vi "MPM_Set_Logging_Paremeter_for_STS.vi"(0 ".NET Reference in":refnum<k24>, 1 "startwave":dbl, 2 "stopwave":dbl, 3 "wavestep":dbl, 4 "speed":dbl, 5 "error in (no error)":errorcluster, 7 "mode":i32(ring) items=["ManualRangeConstant", "ManualRangeSweep", "AutoRangeConstant", "AutoRangeSweep", "Freerun"]) -> (14 "Reference out":refnum<k24>, 19 "error out":errorcluster)   [LabVIEW 2017]
doc: "Sweep parameter setting"
uses:
  D:/test/PDLSTS/LV_PDL_Sample/DLL/InstrumentDLL.dll
  DLL/InstrumentDLL.dll
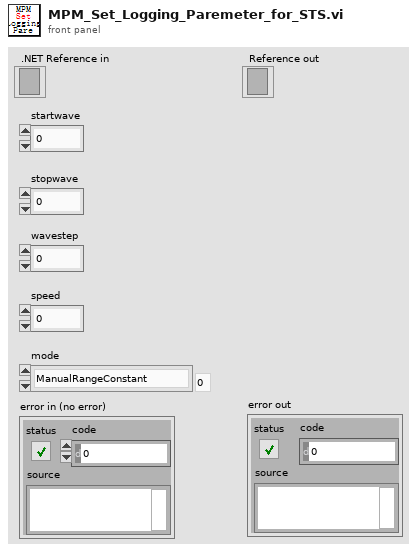
[diagram p1: front panel]
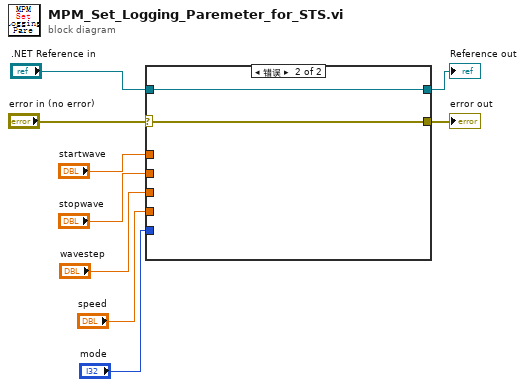
[diagram p0: block diagram]
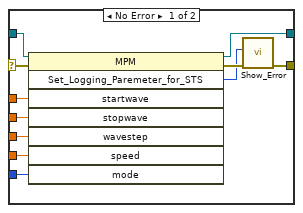
[diagram p2: hidden frame]
diagram:
  n1 = case shown="错误" "error in (no error)" {
    selector: "error in (no error)" -> [w18 w21]
    tunnel: ".NET Reference in" -> [w20 w22]
    tunnel: [w19 w22] -> w8
    tunnel: [w17 w21] -> w6
    tunnel: "startwave" -> [w14 _]
    tunnel: "stopwave" -> [w13 _]
    tunnel: "wavestep" -> [w12 _]
    tunnel: "speed" -> [w11 _]
    tunnel: "mode" -> [w10 _]
    frame No Error {
      n2 = invoke class="MPM" method="Set_Logging_Paremeter_for_STS"(reference=w20, error in=w18, "startwave"=w14, "stopwave"=w13, "wavestep"=w12, "speed"=w11, "mode"=w10) -> (reference out=w19:refnum<k24>, error out=w16:errorcluster, "Set_Logging_Paremeter_for_STS"=w15:i32)  [unwired: 1 in, 5 out]
      n3 = call "Show_Error.vi"("error in (no error)"=w16, "Error"=w15) -> ("error out"=w17:errorcluster)  [unwired: 9 in]
    }
    frame Error {
    }
  }
  "Reference out" <- w8
  "error out" <- w6
